vi "Convert image to real array.vi"(2 "error in":errorcluster, 3 "Image Type":T1 items=["Grayscale (U8)", "Grayscale (I16)", "Grayscale (SGL)", "Complex (CSG)", "RGB (U32)", "HSL (U32)", "RGB (U64)", "Grayscale (U16)"], 4 "x1, y1, x2+1, y2+1 with origin (0, 0)":u16[](array[numeric]), 5 "Image In":T2) -> (0 "error out":errorcluster, 1 "Image Array Out":dbl[][](array[numeric]))   [LabVIEW 2011]
uses:
  <vilib>/vision/Image Controls.llb/IMAQ Image.ctl
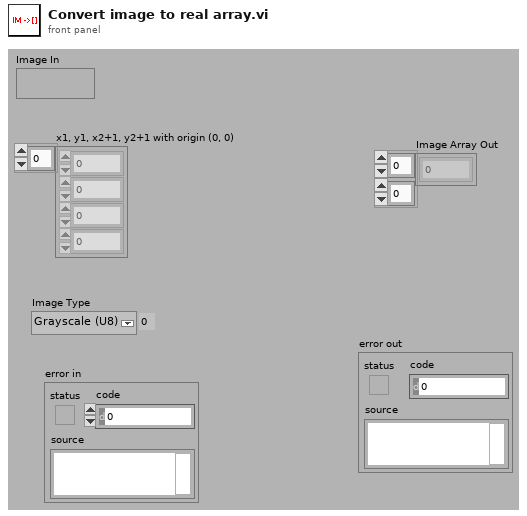
[diagram p1: front panel]
types:
  T1 = typedef "Image Type" = u32
  T2 = typedef "IMAQ Image.ctl" = refnum<image>
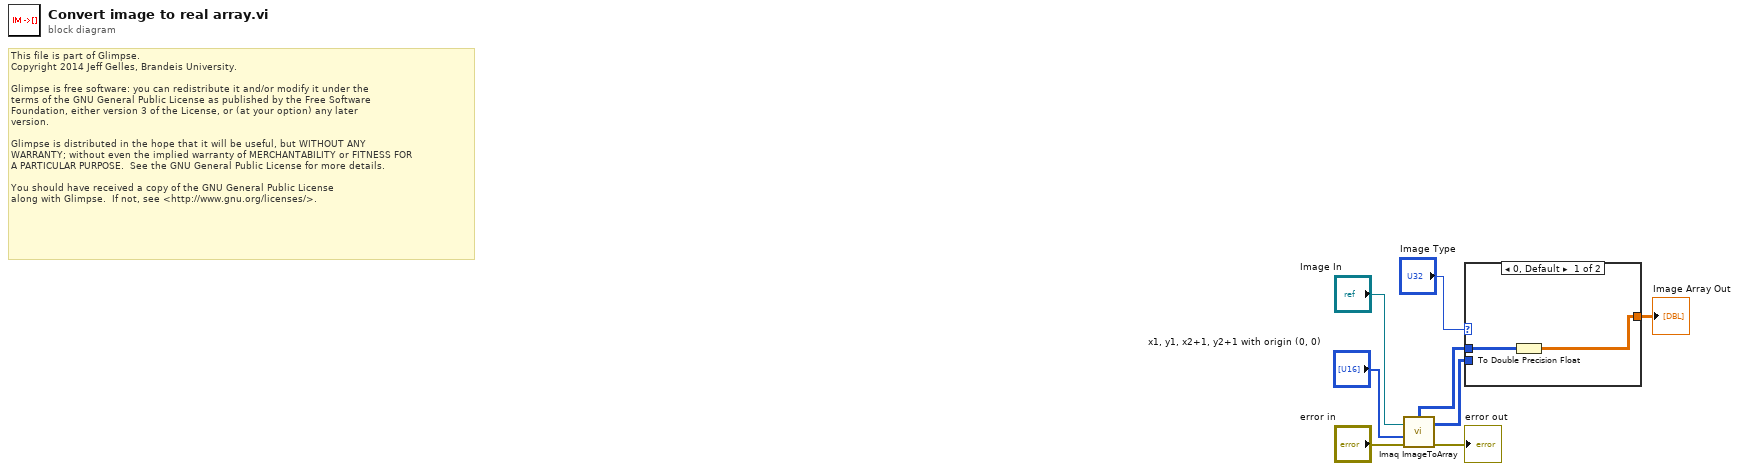
[diagram p0: block diagram]
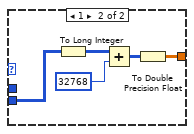
[diagram p2: hidden frame]
diagram:
  # "This file is part of Glimpse. \nCopyright 2014 Jeff Gelles, Brandeis University.    \n\nGlimpse is free software: you can redistribute it and/or modify it under the \nterms of the GNU General Public License as published by the Free Software \nFoundation, either version 3 of the License, or (at your option) any later \nversion.\n\nGlimpse is distributed in the hope that it will be useful, but WITHOUT ANY \nWARRANTY; without even the implied warranty of MERCHANTABILITY or FITNESS FOR \nA PARTICULAR PURPOSE.  See the GNU General Public License for more details.\n\nYou should have received a copy of the GNU General Public License\nalong with Glimpse.  If not, see <http://www.gnu.org/licenses/>."
  n1 = call "Imaq ImageToArray"("error in (no error)"="error in", "Optional Rectangle"="x1, y1, x2+1, y2+1 with origin (0, 0)", "Image"="Image In") -> ("error out"=→"error out":errorcluster, "Image Pixels (U8)"=w6:u8[][], "Image Pixels (I16)"=w7:i16[][])  [unwired: 3 out]
  n2 = case shown="0, Default" "Image Type" {
    tunnel: w6 -> [w10 _]
    tunnel: w7 -> [_ w13]
    tunnel: [w9 w11] -> w8
    frame 0, Default {
      n3 = To Double Precision Float(number=w10) -> (double precision float=w9:dbl[][])
    }
    frame 1 {
      n4 = To Long Integer(number=w13) -> (32bit integer=w14:i32[][])
      n5 = Add(x=w14, y=32768) -> (x+y=w12:i32[][])
      n6 = To Double Precision Float(number=w12) -> (double precision float=w11:dbl[][])
    }
  }
  "Image Array Out" <- w8
